vi "Read Parameter.Hausmodell.vi"(8 "error in (no error)":errorcluster, 11 "Hausmodell in":refnum<class "Hausmodell.lvclass">) -> (0 "error out":errorcluster, 2 "Parameter.Hausmodell":T1={"Bodenfläche [m2]"=0.0, "Raumhöhe [m]"=1.2, "Bodendicke [m]"=0.0, "Hausmaterial Dichte [kg/m3]"=0.0, "Hausmaterial Spez. Wärmekapazität [J/KgK]"=0.0, "U-Wert Boden [W/m2/K]"=0.0, "U-Wert Fenster [W/m2K]"=0.0, "U-Wert Wand/Dach [W/m2K]"=0.0, "Heizrohr Aussenradius [m]"=0.0, "Heizrohr Innenradius [m]"=0.0, "Heizrohr Wärmeleitfähigkeit [W/mK]"=0.0, "Heizrohr Länge pro m2 Bodenfläche [m] "=0.0, "Heizwasser Volumenstrom [m3/h]"=0.0, "Heizwasser Dichte [Kg/m3]"=0.0, "Heizwasser Spez. Wärmekapazität [J/KgK]"=0.0} {"Raumhöhe [m]" format="%#_13g"}, 3 "Hausmodell out":refnum<class "Hausmodell.lvclass">)   [LabVIEW 2016, in "Hausmodell.lvclass"]
uses:
  Hausmodell.lvclass
  Hausmodell.lvclass/Hausmodell.ctl
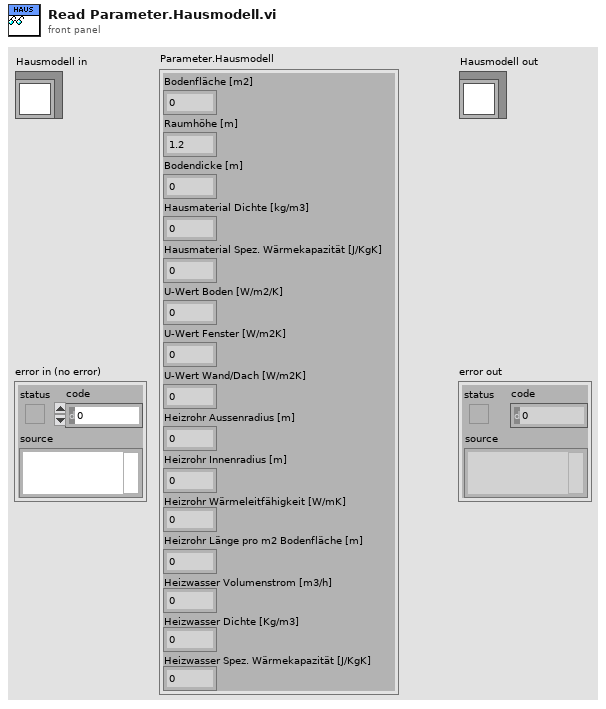
[diagram p1: front panel]
types:
  T1 = cluster{"Bodenfläche [m2]":dbl, "Raumhöhe [m]":dbl, "Bodendicke [m]":dbl, "Hausmaterial Dichte [kg/m3]":dbl, "Hausmaterial Spez. Wärmekapazität [J/KgK]":dbl, "U-Wert Boden [W/m2/K]":dbl, "U-Wert Fenster [W/m2K]":dbl, "U-Wert Wand/Dach [W/m2K]":dbl, "Heizrohr Aussenradius [m]":dbl, "Heizrohr Innenradius [m]":dbl, "Heizrohr Wärmeleitfähigkeit [W/mK]":dbl, "Heizrohr Länge pro m2 Bodenfläche [m] ":dbl, "Heizwasser Volumenstrom [m3/h]":dbl, "Heizwasser Dichte [Kg/m3]":dbl, "Heizwasser Spez. Wärmekapazität [J/KgK]":dbl}
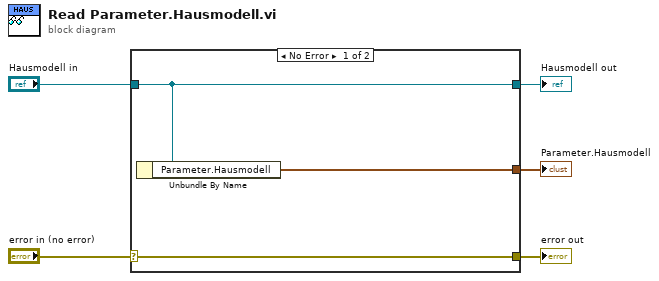
[diagram p0: block diagram]
diagram:
  n1 = case shown="No Error" "error in (no error)" {
    selector: "error in (no error)" -> [w8 w9]
    tunnel: [w8 w9] -> w4
    tunnel: [w7 w10] -> w2
    tunnel: "Hausmodell in" -> [w7 w10]
    tunnel: [w6 _] -> w1
    frame No Error {
      n2 = Unbundle By Name(w7) -> ("Parameter.Hausmodell"=w6:T1)
    }
    frame Error {
    }
  }
  "error out" <- w4
  "Hausmodell out" <- w2
  "Parameter.Hausmodell" <- w1
